vi "Get Target Address.vi"(8 "error in (no error)":errorcluster) -> (0 "error out":errorcluster, 3 "target address":string)   [LabVIEW 2020, in "Logging Loopback.lvclass"]
uses:
  Logging Loopback.lvclass
  <vilib>/NI/VeriStand Custom Device Testing Tools/VeriStandTestUtilities/VeriStandTestUtilities.lvlib
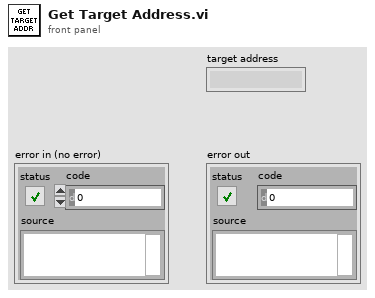
[diagram p1: front panel]
types:
  T1 = typedef "VeriStandTestUtilities.lvlib/TargetsConfiguration.ctl" = cluster{"Supported Targets":cluster{"IP Address / Hostname":string, "Target Platform":T2}[], "Active Configuration":T2}
  T2 = typedef "VeriStandTestUtilities.lvlib/TargetPlatform.ctl" = enum16{"Windows", "Linux64CRIO", "Linux64PXI", "LinuxARM", "PharLap"}
  T3 = cluster{"IP Address / Hostname":string, "Target Platform":T2}[]
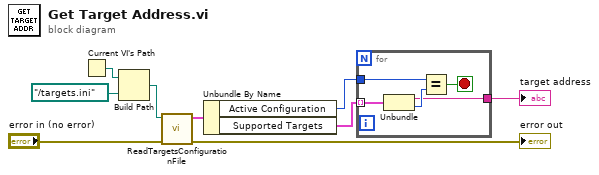
[diagram p0: block diagram]
diagram:
  n1 = Current VI's Path() -> (path=w9:path)
  n2 = Build Path(base path=w9, name or relative path=path "../targets.ini" ("Hardware File Path")) -> (appended path=w7:path)
  n3 = call <vilib>:"ReadTargetsConfigurationFile.vi"("error in (no error)"="error in (no error)", "targets.ini file"=w7) -> ("error out"=→"error out":errorcluster, "Targets Configuration"=w8:T1)  [unwired: 8 in]
  n4 = Unbundle By Name(w8) -> ("Active Configuration"=w2:T2, "Supported Targets"=w3:T3)
  n5 = for {
    tunnel: w3 -> [w14] mode=indexing
    tunnel: w2 -> [w13]
    tunnel: [w10] -> w1
    stop <- w12 stop-if-true
    n6 = Unbundle(w14) -> ("IP Address / Hostname"=w10:string, "Target Platform"=w11:T2)
    n7 = Equal?(x=w13, y=w11) -> (x = y?=w12:bool)
  }
  "target address" <- w1
